vi "Insight_R_Frequency_Step.vi"(8 "error in (no error)":errorcluster, 11 "telnet connection":T1) -> (0 "error out":errorcluster, 1 "response data":string, 2 "Optical Frequency Step (GHz)":dbl format="%.3g", 3 "telnet  connection out":T1)   [LabVIEW 2011]
doc: "Insight Photonic Solutions\n\nThis VI reads the optical frequency step, in GHz, between valid points in the laser sweep.\n\nver 1.0 - original release\nver1.1 - added Buffer Output\nver3.2 - updated parser to accept responses from Atlas 3.1 and earlier or Atlas 3.2 and later."
uses:
  Telnet Session.ctl
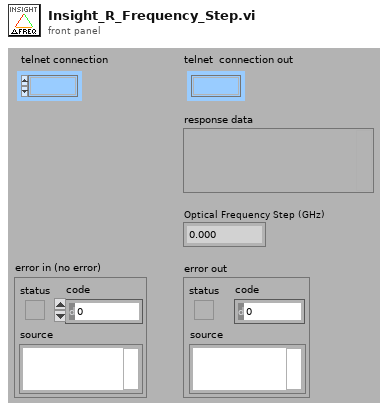
[diagram p1: front panel]
types:
  T1 = typedef "Telnet Session.ctl" = refnum<k1>
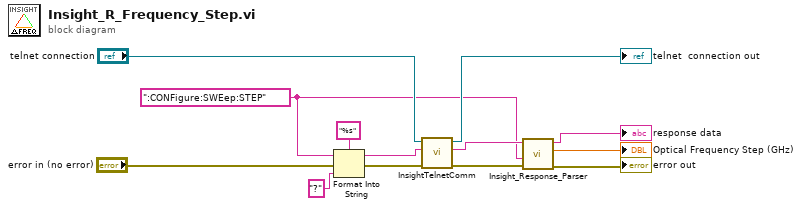
[diagram p0: block diagram]
diagram:
  w1 = ":CONFigure:SWEep:STEP" ("String")
  n1 = Format Into String(format string="%s", initial string=w1, error in="error in (no error)", "?" ("input 1")) -> (resulting string=w7:string, error out=w10:errorcluster)
  n2 = call "InsightTelnetComm.vi"("error in"=w10, "write buffer (\"\")"=w7, "telnet connection"="telnet connection") -> ("error out"=w2:errorcluster, "response data"=w6:string, "telnet  connection out"=→"telnet  connection out":T1)  [unwired: 4 in]
  n3 = call "Insight_Response_Parser.vi"("error in (no error)"=w2, "Command String"=w1, "Laser Response In"=w6) -> ("error out"=→"error out":errorcluster, "Value"=→"Optical Frequency Step (GHz)":dbl, "Laser Response Out"=→"response data":string)  [unwired: 6 in]
